vi "Write Monitor File.vi"(8 "error in (no error)":errorcluster, 9 "Open plot":bool, 10 "Monitor File":path, 11 "Monitor-Pulse in":refnum<class "Monitor-Pulse.lvclass">) -> (0 "error out":errorcluster, 3 "Monitor-Pulse out":refnum<class "Monitor-Pulse.lvclass">)   [LabVIEW 2016, in "Monitor-Pulse.lvclass"]
uses:
  Monitor-Pulse.lvclass
  Measure_core/Plots/Plot types.ctl
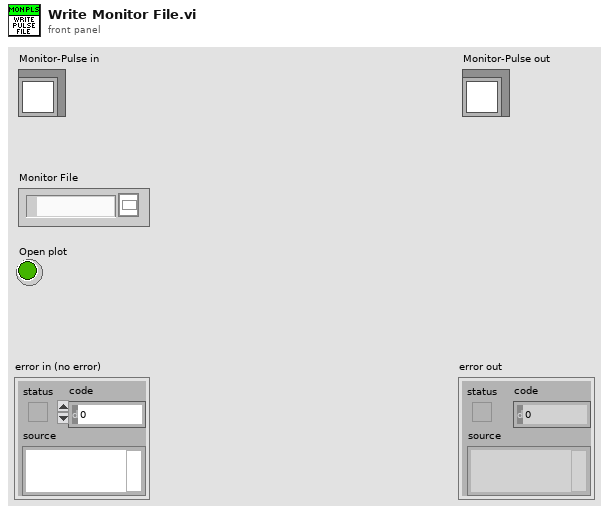
[diagram p1: front panel]
types:
  T1 = typedef "Plot types.ctl" = enum16{"Waveform Plot", "XY Plot", "Full XY"}
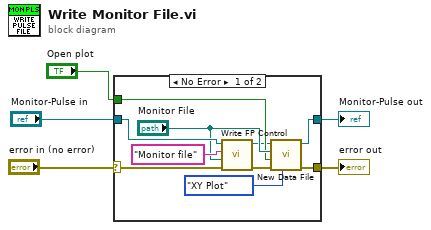
[diagram p0: block diagram]
diagram:
  n1 = case shown="No Error" "error in (no error)" {
    selector: "error in (no error)" -> [w13 w17]
    tunnel: [w6 w17] -> w4
    tunnel: [w8 w16] -> w2
    tunnel: "Monitor-Pulse in" -> [w15 w16]
    tunnel: "Open plot" -> [w10 _]
    frame No Error {
      n2 = call-dynamic "Write FP Control.vi"("error in (no error)"=w13, "Control Value"="Monitor File", "Control Name"="Monitor file", "Measure Object in"=w15) -> ("error out"=w7:errorcluster, "Measure Object out"=w9:refnum<class "Monitor-Pulse.lvclass">)  [unwired: 6 in]
      n3 = call-dynamic "New Data File.vi"("Plot type"=Plot_types."XY Plot", "error in (no error)"=w7, "New plot if not open"=w10, "File"="Monitor File", "Application Controller in"=w9) -> ("error out"=w6:errorcluster, "Application Controller out"=w8:refnum<class "Monitor-Pulse.lvclass">)  [unwired: 5 in]
    }
    frame Error {
    }
  }
  "error out" <- w4
  "Monitor-Pulse out" <- w2
